vi "Read Recording From Disk.vi"(8 "error in (no error)":errorcluster, 11 "File Path":path=path "sample.wav") -> (0 "error out":errorcluster, 3 "Recorded Sound":refnum<class "Recorded Sound.lvclass">)   [LabVIEW 2010, in "Recorded Sound.lvclass"]
uses:
  Recorded Sound.lvclass
  Recorded Sound.lvclass/Recorded Sound.ctl
  <vilib>/sound2/lvsound2.llb/Sound File Read Open.vi
  <vilib>/sound2/lvsound2.llb/Sound File Read (DBL).vi
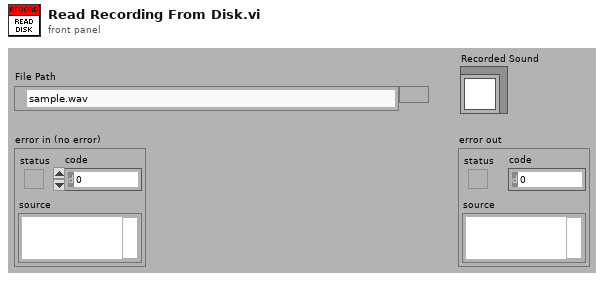
[diagram p1: front panel]
types:
  T1 = typedef "Sound File Refnum.ctl" = refnum<file>
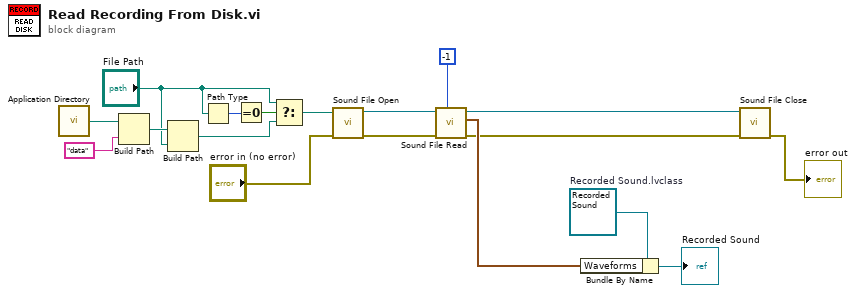
[diagram p0: block diagram]
diagram:
  w14 = refnum<class "Recorded Sound.lvclass"> refnum  # Recorded Sound.lvclass
  n1 = call <vilib>:"Application Directory.vi"() -> ("Application Directory"=w5:path)
  n2 = Build Path(base path=w5, name or relative path="data") -> (appended path=w6:path)
  n3 = Build Path(base path=w6, name or relative path="File Path") -> (appended path=w8:path)
  n4 = Path Type(1:"File Path") -> (0:w10:i16)
  n5 = Equal To 0?(x=w10) -> (x = 0?=w9:bool)
  n6 = Select(t="File Path", s=w9, f=w8) -> (s? t:f=w7:path)
  n7 = call-poly <vilib>:"Sound File Open.vi"("error in (no error)"="error in (no error)", "path"=w7) -> ("error out"=w15:errorcluster, "sound file refnum"=w17:T1)  [unwired: 8 in]
  n8 = call-poly <vilib>:"Sound File Read.vi"("number of samples/ch (-1: all)"=-1 ("Number of Samples/Iteration"), "error in (no error)"=w15, "sound file refnum"=w17) -> ("error out"=w1:errorcluster, "data"=w2:waveform(dbl)[], "sound file refnum out"=w18:T1)  [unwired: 4 in, 2 out]
  n9 = Bundle By Name(cluster=w14, "Waveforms"=w2) -> (→"Recorded Sound":refnum<class "Recorded Sound.lvclass">)
  n10 = call <vilib>:"Sound File Close.vi"("error in (no error)"=w1, "sound file refnum"=w18) -> ("error out"=→"error out":errorcluster)  [unwired: 9 in]
